vi "Tower_lamp.vi"(7 "FCT/EOL":bool, 9 "queue IN":refnum<queue>, 10 "DOs":bool[](array[boolean])=[TRUE, FALSE, FALSE, FALSE], 11 "Relay_Channel_OUT":T1[](array[typedef])) -> ()   [LabVIEW 2024, in "Relay_Module.lvlib"]
uses:
  Relay_Module.lvlib
  Relay_Enum_OUT.ctl
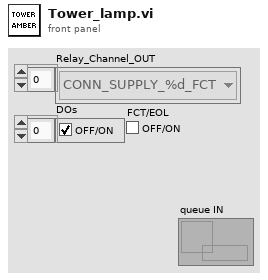
[diagram p1: front panel]
types:
  T1 = typedef "Relay_Module.lvlib/Relay_Enum_OUT.ctl" = enum16{"CONN_SUPPLY_%d_FCT", "HB_CONN_%d_FCT", "L_IND_CONN_%d_FCT", "R_IND_CONN_%d_FCT", "SW1_%d_FCT", "SW2_%d_FCT", "CAN_H_%d_FCT", "CAN_L_%d_FCT", "CYLINDER_ON/OFF_%d_FCT", "SPARE_1_%d_FCT", "SPARE_2_%d_FCT", "Tower Red", "Tower Amber", "Tower Green", "Tower Buzzer", "SLIMRELAY_DUT_%d_FCT", "GND_DMM_%d_EOL", "CAN_H_RES_%d_EOL", "CAN_L_RES_%d_EOL", "L_IND_RES_%d_EOL", "R_IND_RES_%d_EOL", "HB_CONN_DMM_%d_EOL", "14V_RES_%d_EOL", "CAN_L_(DMM-)_%d_EOL", "CAN_H_%d_EOL", "CAN_L_%d_EOL", "14V_%d_EOL", "GND_%d_EOL", "HB_CONN_%d_EOL", "L_IND_%d_EOL", "R_IND_%d_EOL", "CYLINDER_DUT_%d_EOL", "CYL_PB_1_%d_EOL", "CYL_PB_2_%d_EOL", "DUT_PASS_%d_EOL", "DUT_FAIL_%d_EOL", "SPARE1_%d_EOL", "Tower Red_EOL", "Tower Amber_EOL", "Tower Green_EOL", "Tower Buzzer_EOL"}
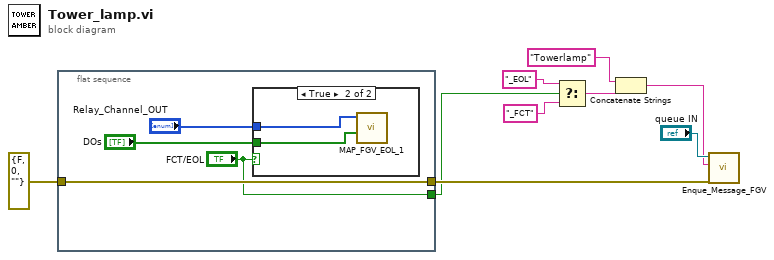
[diagram p0: block diagram]
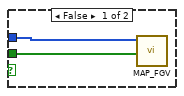
[diagram p2: hidden frame]
diagram:
  n1 = flat-sequence {
    tunnel: errorcluster {"status"=FALSE, "code"=0, "source"=""} ("error out") -> [w12]
    tunnel: [w12] -> w9
    tunnel: ["FCT/EOL"] -> w6
    frame #0 {
      n2 = case shown="True" "FCT/EOL" {
        tunnel: "DOs" -> [w15 w16]
        tunnel: "Relay_Channel_OUT" -> [w14 w17]
        frame False {
          n3 = call "MAP_FGV.vi"("DOs"=w15, "Relay_Channel_Out"=w14) -> ()  [unwired: 7 in, 3 out]
        }
        frame True {
          n4 = call "MAP_FGV_EOL_1.vi"("DOs"=w16, "Relay_Channel_Out"=w17) -> ()  [unwired: 7 in, 3 out]
        }
      }
    }
  }
  n5 = Select(t="_EOL", s=w6, f="_FCT") -> (s? t:f=w5:string)
  n6 = Concatenate Strings("Towerlamp", w5) -> (w1:string)
  n7 = call "Enque_Message_FGV.vi"("error in (no error)"=w9, "Message"=w1, "queue IN"="queue IN") -> ()  [unwired: 8 in, 1 out]
